vi "Inline or forked test vi.vi"() -> ()   [LabVIEW 2017]
panel:
  out "Numeric 2":i32
  in  "Numeric":i32
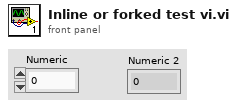
[diagram p1: front panel]
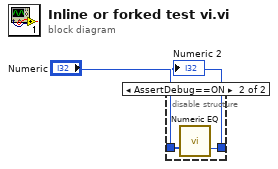
[diagram p0: block diagram]
diagram:
  n1 = disable-structure "AssertVI_CDS" shown="AssertDebug==ON" {
    disable-tunnel: [w3 w4] -> w1
    disable-tunnel: "Numeric" -> [w3 w4]
    frame condition #0 {
    }
    frame condition #1 (active) {
      # "Assert"
      n2 = call "Numeric EQ.vi"("Data In"=w4) -> ()  [unwired: 10 in, 1 out]
    }
  }
  "Numeric 2" <- w1
